vi "AlazarResetTimeStamp.vi"(3 "error in (no error)":errorcluster, 4 "Option":u32(ring) items=["Reset First Time Only", "Reset Always"], 5 "Handle":u64) -> (0 "error out":errorcluster, 1 "Return Code":u32, 2 "Handle":u64)   [LabVIEW 2018]
doc: "Control record timestamp counter resets."
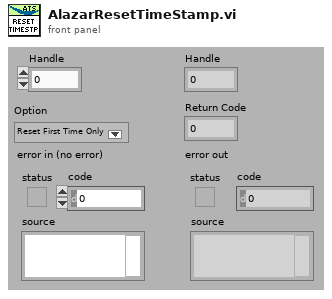
[diagram p1: front panel]
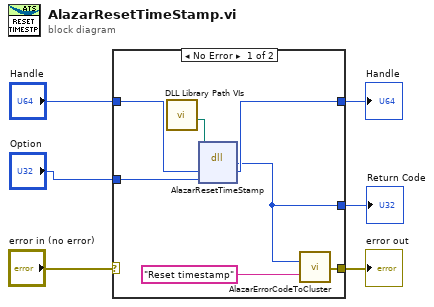
[diagram p0: block diagram]
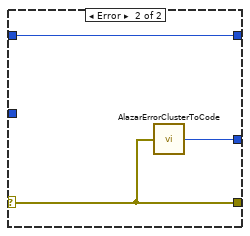
[diagram p2: hidden frame]
diagram:
  n1 = case shown="No Error" "error in (no error)" {
    selector: "error in (no error)" -> [_ w16]
    tunnel: [w10 w16] -> w5
    tunnel: [w9 w15] -> w4
    tunnel: "Handle" -> [w13 w14]
    tunnel: [w12 w14] -> w2
    tunnel: "Option" -> [w11 _]
    frame No Error {
      n2 = call "DLL Library Path VIs.vi"() -> ("Alazar"=w7:path)  [unwired: 9 in, 2 out]
      n3 = dll-call lib="C:/Project/SerialSectOCT - FFT GPU/SerialSectOCT/Labview Software/DLL/ATSApi.dll" fn="AlazarResetTimeStamp"(path in=w7, "handle"=w13, "option"=w11) -> ("return type"=w9:u32, "handle"=w12:u64)  [unwired: 3 in, 2 out]
      n4 = call "AlazarErrorCodeToCluster.vi"("Message"="Reset timestamp", "Error Code"=w9) -> ("error out"=w10:errorcluster)
    }
    frame Error {
      n5 = call "AlazarErrorClusterToCode.vi"("error in (no error)"=w16) -> ("Error Code"=w15:u32)
    }
  }
  "Handle" <- w2
  "error out" <- w5
  "Return Code" <- w4
